vi "Actor Core.vi"(8 "error in":errorcluster, 11 "PriceData in":refnum<class "PriceData.lvclass">) -> (0 "error out":errorcluster, 3 "Actor out":refnum<class "Actor.lvclass">)   [LabVIEW 2018, in "PriceData Actor.lvlib" / "PriceData.lvclass"]
doc: "(<B>Filename</B>: Actor Framework.lvlib:Actor.lvclass:Actor Core.vi)\n\nReceives messages to the actor, reacts to them, and initiates any error handling that may shut the actor down.\n\nDescendant classes may override this VI to append parallel tasks for the actor to complete while it handles messages. Overrides use the Call Parent Method node."
uses:
  PriceData.lvclass
  C:/Users/Administrator/Desktop/LabVIEW EMS/EMS Generic Actor/EMS Generic/EMS Generic.lvclass
  <vilib>/ActorFramework/Actor/Actor.lvclass
  EMS Generic Actor/EMS Generic/EMS Generic.lvclass/EMS Generic.ctl
  <vilib>/ORNL/CSEISMIC DDS/CSEISMIC DDS Base/CSEISMIC DDS.lvclass/CSEISMIC DDS.ctl
  <vilib>/ORNL/CSEISMIC DDS/CSEISMIC DDS Base/Accessors/Write DDS Reference.vi
  <vilib>/ORNL/CSEISMIC DDS/CSEISMIC DDS Base/Accessors/Read DDS Reference.vi
  <vilib>/ORNL/CSEISMIC DDS/DDS Reader/DDS Reader.lvclass
  C:/Program Files (x86)/National Instruments/LabVIEW 2018/vi.lib/ORNL/CSEISMIC DDS/CSEISMIC DDS Base/CSEISMIC DDS.lvclass
  <vilib>/ORNL/CSEISMIC DDS/CSEISMIC DDS Base/Error Handler.vi
  Device DDS Communications Framework/Device DDS Communications/Device DDS Communications.lvclass
  EMS Generic Actor/EMS Generic/EMS Generic.lvclass
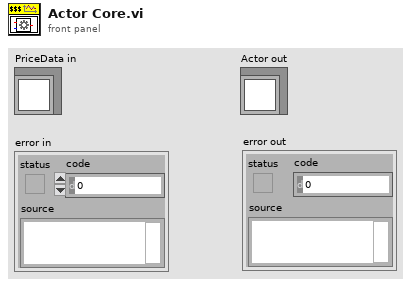
[diagram p1: front panel]
types:
  T1 = typedef "CSEISMIC DDS.lvlib/CSEISMIC DDS.lvclass/DeviceID.ctl" = string
  T2 = typedef "CSEISMIC DDS.lvlib/CSEISMIC DDS.lvclass/PriceData_RealTime.ctl" = cluster{"DeviceID":T1, "t0":dbl, "dt":dbl, "Price":dbl[]}
  T3 = typedef "LVDDS_library.lvlib/DDS Sample Info.ctl" = cluster{"DDS_SampleStateKind":enum32{"DDS_INVALID_SAMPLE_STATE", "DDS_READ_SAMPLE_STATE", "DDS_NOT_READ_SAMPLE_STATE"}, "DDS_ViewStateKind":enum32{"DDS_INVALID_SAMPLE_STATE", "DDS_NEW_VIEW_STATE", "DDS_NOT_NEW_VIEW_STATE"}, "DDS_InstanceStateKind":enum32{"DDS_INVALID_STATE", "DDS_ALIVE_INSTANCE_STATE", "DDS_NOT_ALIVE_DISPOSED_INSTANCE_STATE", "", "DDS_NOT_ALIVE_NO_WRITERS_INSTANCE_STATE"}, "sec":i32, "nanosec":u32, "valid_data":bool}
  T4 = typedef "CSEISMIC DDS.lvlib/CSEISMIC DDS.lvclass/PriceData_Demand.ctl" = cluster{"DeviceID":T1, "DemandCharge ($/kWh)":dbl, "Duration (hours)":dbl}
  T5 = typedef "CSEISMIC DDS.lvlib/CSEISMIC DDS.lvclass/PriceData_Energy.ctl" = cluster{"DeviceID":T1, "EnergyCharge ($/kWh)":dbl}
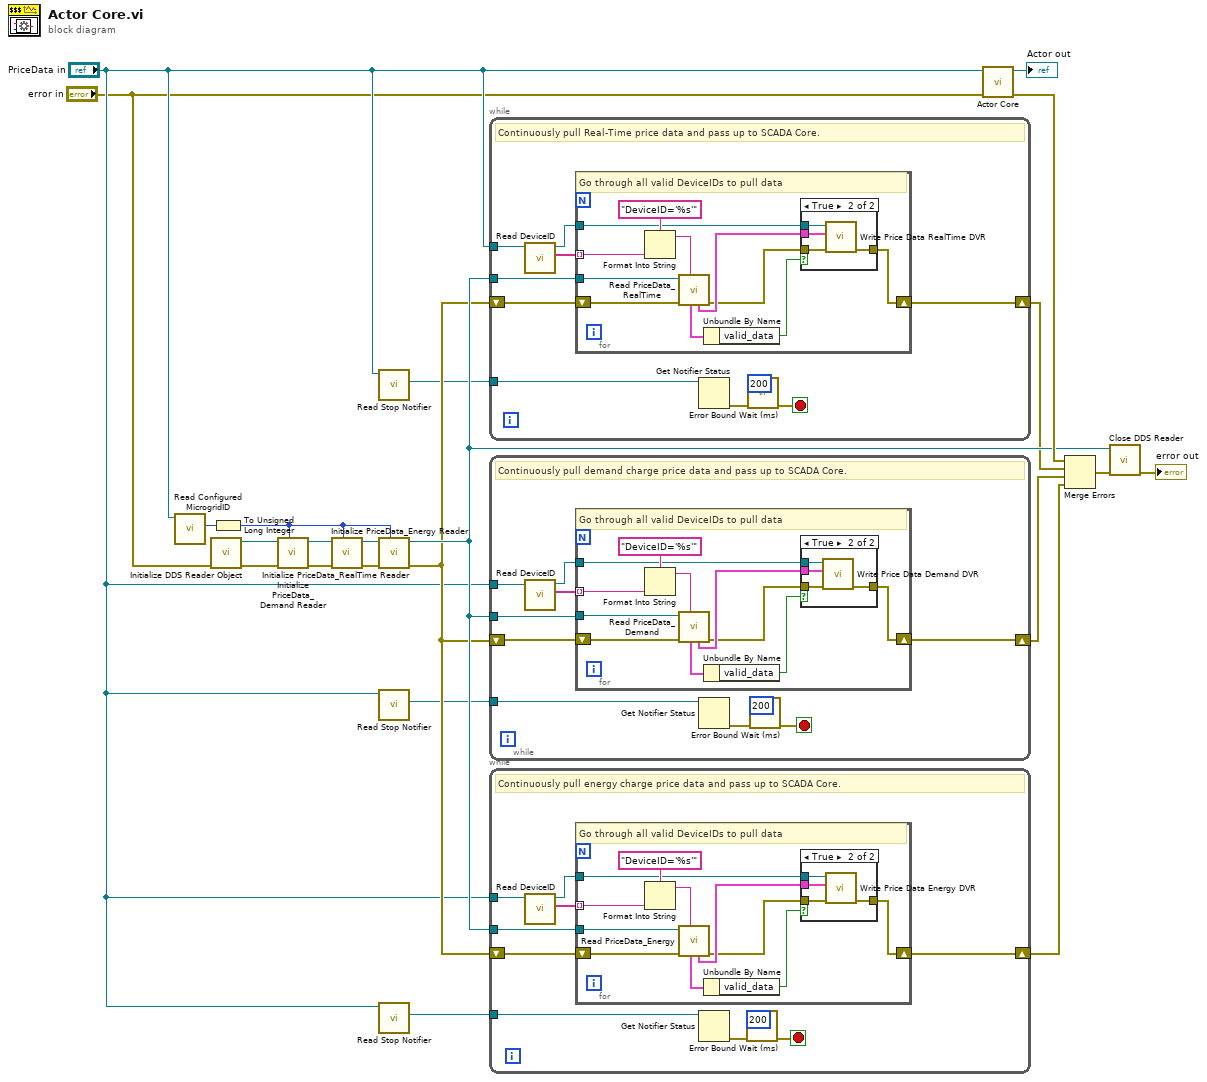
[diagram p0: block diagram]
diagram:
  n1 = call "Read Configured MicrogridID.vi"("EMS Generic in"="PriceData in") -> ("Microgrid ID"=w22:u8)  [unwired: 8 in, 2 out]
  n2 = call <vilib>:"Initialize DDS Reader Object.vi"("error in"="error in") -> ("error out"=w18:errorcluster, "DDS Reader out"=w17:refnum<class "DDS Reader.lvclass">)  [unwired: 9 in]
  n3 = To Unsigned Long Integer(number=w22) -> (unsigned 32bit integer=w10:u32)
  n4 = call <vilib>:"Initialize PriceData_Demand Reader.vi"("MicrogridID"=w10, "error in"=w18, "DDS Reader in"=w17) -> ("error out"=w19:errorcluster, "DDS Reader out"=w16:refnum<class "DDS Reader.lvclass">)  [unwired: 7 in]
  n5 = call <vilib>:"Initialize PriceData_Energy Reader.vi"("MicrogridID"=w10, "error in"=w19, "DDS Reader in"=w16) -> ("error out"=w12:errorcluster, "DDS Reader out"=w14:refnum<class "DDS Reader.lvclass">)  [unwired: 7 in]
  n6 = call "Read Stop Notifier.vi"("EMS Generic in"="PriceData in") -> ("stop"=w9:refnum<notifier>)  [unwired: 9 in, 1 out]
  n7 = call <vilib>:"Initialize PriceData_RealTime Reader.vi"("MicrogridID"=w10, "error in"=w12, "DDS Reader in"=w14) -> ("error out"=w11:errorcluster, "DDS Reader out"=w13:refnum<class "DDS Reader.lvclass">)  [unwired: 7 in]
  n8 = call "Read Stop Notifier.vi"("EMS Generic in"="PriceData in") -> ("stop"=w1:refnum<notifier>)  [unwired: 9 in, 1 out]
  n9 = call "Read Stop Notifier.vi"("EMS Generic in"="PriceData in") -> ("stop"=w15:refnum<notifier>)  [unwired: 9 in, 1 out]
  n10 = while {
    tunnel: w9 -> [w32]
    shift-right: [w31] -> w6
    shift-left: w11 -> [w28]
    tunnel: "PriceData in" -> [w29]
    tunnel: w13 -> [w27]
    stop <- w26 stop-if-true
    # "Continuously pull Real-Time price data and pass up to SCADA Core."
    n11 = call-dynamic "Read DeviceID.vi"("Device DDS Communications in"=w29) -> ("DeviceID"=w24:T1[], "Device DDS Communications out"=w23:refnum<class "PriceData.lvclass">)  [unwired: 9 in]
    n12 = for {
      shift-right: [w33] -> w31
      shift-left: w28 -> [w42]
      tunnel: w24 -> [w40] mode=indexing
      tunnel: w23 -> [w35]
      tunnel: w27 -> [w43]
      # "Go through all valid DeviceIDs to pull data"
      n13 = Format Into String(format string="DeviceID='%s'", w40) -> (resulting string=w39:string)  [unwired: 2 in, 1 out]
      n14 = call <vilib>:"Read PriceData_RealTime.vi"("Query condition"=w39, "error in"=w42, "DDS Reader in"=w43) -> ("error out"=w34:errorcluster, "data"=w36:T2, "DDS Sample Info"=w38:T3)  [unwired: 5 in, 1 out]
      n15 = Unbundle By Name(w38) -> ("valid_data"=w37:bool)
      n16 = case shown="True" w37 {
        tunnel: w36 -> [_ w48]
        tunnel: w35 -> [_ w47]
        tunnel: w34 -> [w44 w46]
        tunnel: [w44 w45] -> w33
        frame False {
        }
        frame True {
          n17 = call "Write Price Data RealTime DVR.vi"("error in"=w46, "PriceData_RealTime"=w48, "EMS Generic in"=w47) -> ("error out"=w45:errorcluster)  [unwired: 7 in, 1 out]
        }
      }
    }
    n18 = Get Notifier Status(notifier=w32) -> (error out=w30:errorcluster)  [unwired: 1 in, 4 out]
    n19 = call "Error Bound Wait (ms).vi"("milliseconds to wait (100)"=u32 200 ("milliseconds to wait"), "error in"=w30) -> ("error out"=w26:errorcluster)  [unwired: 9 in]
  }
  n20 = while {
    tunnel: w1 -> [w58]
    shift-right: [w51] -> w5
    shift-left: w11 -> [w54]
    tunnel: "PriceData in" -> [w52]
    tunnel: w13 -> [w53]
    stop <- w50 stop-if-true
    # "Continuously pull demand charge price data and pass up to SCADA Core."
    n21 = call-dynamic "Read DeviceID.vi"("Device DDS Communications in"=w52) -> ("DeviceID"=w55:T1[], "Device DDS Communications out"=w56:refnum<class "PriceData.lvclass">)  [unwired: 9 in]
    n22 = for {
      shift-right: [w59] -> w51
      shift-left: w54 -> [w68]
      tunnel: w55 -> [w66] mode=indexing
      tunnel: w56 -> [w61]
      tunnel: w53 -> [w69]
      # "Go through all valid DeviceIDs to pull data"
      n23 = Format Into String(format string="DeviceID='%s'", w66) -> (resulting string=w65:string)  [unwired: 2 in, 1 out]
      n24 = call <vilib>:"Read PriceData_Demand.vi"("Query condition"=w65, "error in"=w68, "DDS Reader in"=w69) -> ("error out"=w60:errorcluster, "data"=w62:T4, "DDS Sample Info"=w64:T3)  [unwired: 5 in, 1 out]
      n25 = Unbundle By Name(w64) -> ("valid_data"=w63:bool)
      n26 = case shown="True" w63 {
        tunnel: w62 -> [_ w71]
        tunnel: w61 -> [_ w72]
        tunnel: w60 -> [w70 w74]
        tunnel: [w70 w73] -> w59
        frame False {
        }
        frame True {
          n27 = call "Write Price Data Demand DVR.vi"("error in"=w74, "PriceData_Demand"=w71, "EMS Generic in"=w72) -> ("error out"=w73:errorcluster)  [unwired: 7 in, 1 out]
        }
      }
    }
    n28 = Get Notifier Status(notifier=w58) -> (error out=w57:errorcluster)  [unwired: 1 in, 4 out]
    n29 = call "Error Bound Wait (ms).vi"("milliseconds to wait (100)"=u32 200 ("milliseconds to wait"), "error in"=w57) -> ("error out"=w50:errorcluster)  [unwired: 9 in]
  }
  n30 = while {
    tunnel: w15 -> [w84]
    shift-right: [w77] -> w4
    shift-left: w11 -> [w78]
    tunnel: w13 -> [w79]
    tunnel: "PriceData in" -> [w80]
    stop <- w76 stop-if-true
    # "Continuously pull energy charge price data and pass up to SCADA Core."
    n31 = call-dynamic "Read DeviceID.vi"("Device DDS Communications in"=w80) -> ("DeviceID"=w82:T1[], "Device DDS Communications out"=w81:refnum<class "PriceData.lvclass">)  [unwired: 9 in]
    n32 = for {
      shift-right: [w85] -> w77
      shift-left: w78 -> [w94]
      tunnel: w82 -> [w92] mode=indexing
      tunnel: w81 -> [w87]
      tunnel: w79 -> [w95]
      # "Go through all valid DeviceIDs to pull data"
      n33 = Format Into String(format string="DeviceID='%s'", w92) -> (resulting string=w91:string)  [unwired: 2 in, 1 out]
      n34 = call <vilib>:"Read PriceData_Energy.vi"("Query condition"=w91, "error in"=w94, "DDS Reader in"=w95) -> ("error out"=w86:errorcluster, "data"=w88:T5, "DDS Sample Info"=w90:T3)  [unwired: 5 in, 1 out]
      n35 = Unbundle By Name(w90) -> ("valid_data"=w89:bool)
      n36 = case shown="True" w89 {
        tunnel: w88 -> [_ w97]
        tunnel: w87 -> [_ w98]
        tunnel: w86 -> [w96 w100]
        tunnel: [w96 w99] -> w85
        frame False {
        }
        frame True {
          n37 = call "Write Price Data Energy DVR.vi"("error in"=w100, "PriceData_Energy"=w97, "EMS Generic in"=w98) -> ("error out"=w99:errorcluster)  [unwired: 7 in, 1 out]
        }
      }
    }
    n38 = Get Notifier Status(notifier=w84) -> (error out=w83:errorcluster)  [unwired: 1 in, 4 out]
    n39 = call "Error Bound Wait (ms).vi"("milliseconds to wait (100)"=u32 200 ("milliseconds to wait"), "error in"=w83) -> ("error out"=w76:errorcluster)  [unwired: 9 in]
  }
  n40 = call-parent "Actor Core.vi"("error in"="error in", "Actor in"="PriceData in") -> ("error out"=w20:errorcluster, "Actor out"=→"Actor out":refnum<class "Actor.lvclass">)  [unwired: 8 in]
  n41 = Merge Errors(w20, w6, w5, w4) -> (w3:errorcluster)
  n42 = call <vilib>:"Close DDS Reader.vi"("error in"=w3, "DDS Reader in"=w13) -> ("error out"=→"error out":errorcluster)  [unwired: 9 in]
